vi "PR_SPOUT.vi"(7 "QC result":string="NG,", 8 "error in (no error)":errorcluster, 9 "[workplace_id]":i16=2, 10 "當前工位資料":cluster{"barcode R":string, "barcode L":string}, 11 "DBlink":string="Driver={ODBC Driver 17 for SQL Server};Server=localhost\\SQLEXPRESS;Database=ZDX201;UID=labview;PWD=Dsa@54137926") -> (0 "error out":errorcluster)   [LabVIEW 2019]
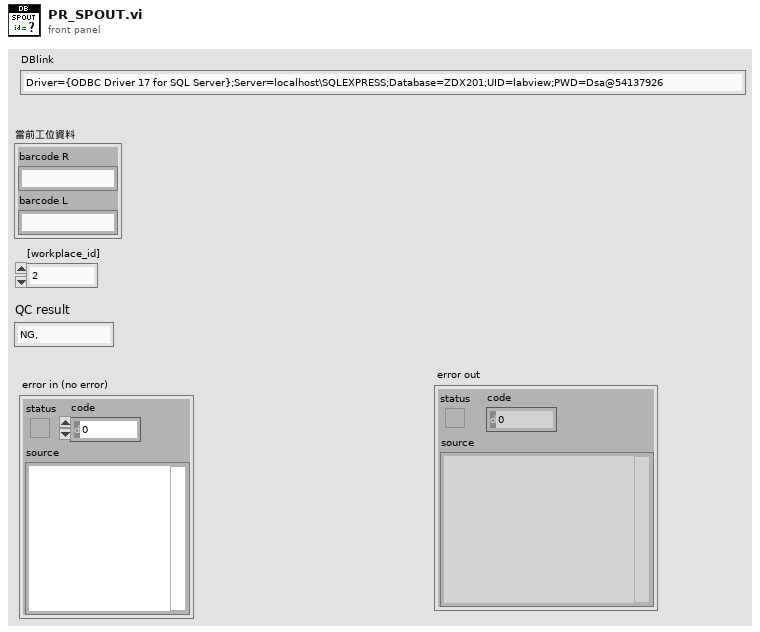
[diagram p1: front panel]
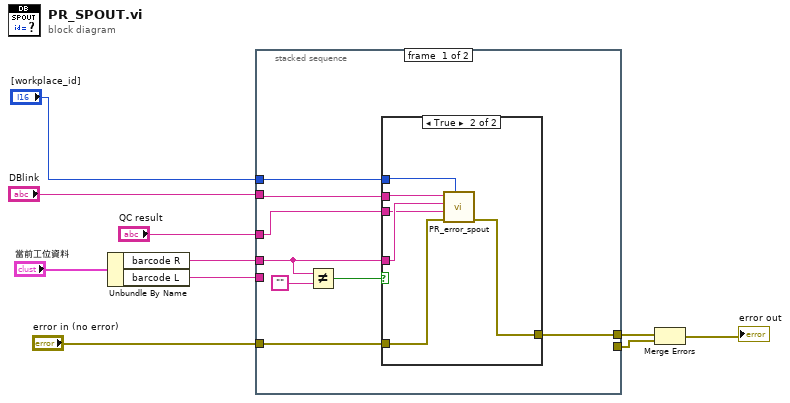
[diagram p0: block diagram]
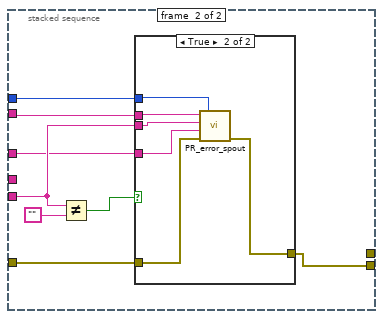
[diagram p3: hidden frame]
diagram:
  n1 = Unbundle By Name("當前工位資料") -> ("barcode R"=w6:string, "barcode L"=w5:string)
  n2 = stacked-sequence {
    tunnel: "[workplace_id]" -> [w18 w33]
    tunnel: "DBlink" -> [w17 w32]
    tunnel: "error in (no error)" -> [w16 w31]
    tunnel: w6 -> [w12 _]
    tunnel: w5 -> [_ w27]
    tunnel: [_ w28] -> w4
    tunnel: [w13 _] -> w3
    tunnel: "QC result" -> [w11 w26]
    frame #0 {
      n3 = Not Equal?(x=w12, y="") -> (x != y?=w14:bool)
      n4 = case shown="True" w14 {
        tunnel: w18 -> [_ w22]
        tunnel: w17 -> [_ w25]
        tunnel: w16 -> [w19 w23]
        tunnel: [w19 w21] -> w13
        tunnel: w12 -> [_ w24]
        tunnel: w11 -> [_ w20]
        frame False {
        }
        frame True {
          n5 = call "PR_error_spout .vi"("[workplace_id]"=w22, "error in (no error)"=w23, "QC result"=w20, "barcode"=w24, "DBlink"=w25) -> ("error out"=w21:errorcluster)  [unwired: 6 in]
        }
      }
    }
    frame #1 {
      n6 = Not Equal?(x=w27, y="") -> (x != y?=w29:bool)
      n7 = case shown="True" w29 {
        tunnel: w33 -> [_ w40]
        tunnel: w32 -> [_ w39]
        tunnel: w31 -> [w34 w37]
        tunnel: [w34 w36] -> w28
        tunnel: w27 -> [_ w38]
        tunnel: w26 -> [_ w35]
        frame False {
        }
        frame True {
          n8 = call "PR_error_spout .vi"("[workplace_id]"=w40, "error in (no error)"=w37, "QC result"=w35, "barcode"=w38, "DBlink"=w39) -> ("error out"=w36:errorcluster)  [unwired: 6 in]
        }
      }
    }
  }
  n9 = Merge Errors(w3, w4) -> (→"error out":errorcluster)
